vi "Boolean Counter.vi"(1 "Input Boolean":bool, 2 "Min of array which must be true":i16=5, 3 "Array Size":i32=5) -> (0 "Output Boolean":bool)   [LabVIEW 2015]
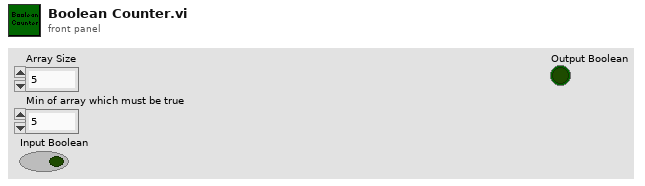
[diagram p1: front panel]
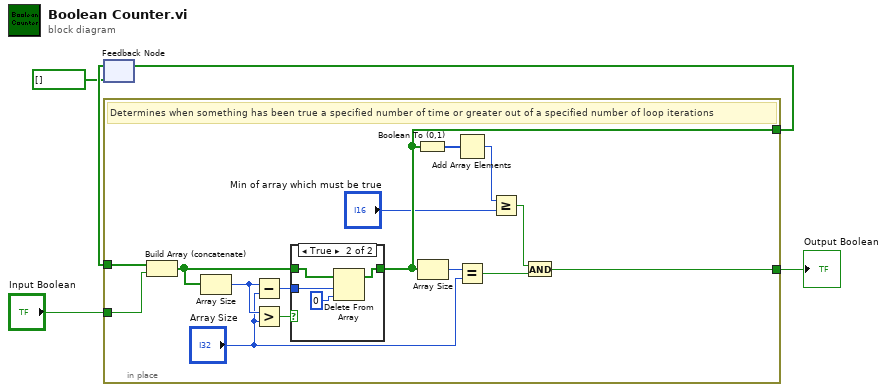
[diagram p0: block diagram]
diagram:
  n1 = feedback #1(bool[] []) -> (w4:bool[])
  n2 = in-place {
    in-place-border: w4 -> [w20]
    in-place-border: [w10] -> w5
    in-place-border: [w12] -> w1
    in-place-border: "Input Boolean" -> [w11]
    # "Determines when something has been true a specified number of time or greater out of a specified number of loop iterations"
    n3 = Build Array (concatenate)(w20, w11) -> (w19:bool[])
    n4 = Array Size(array=w19) -> (size(s)=w17:i32)
    n5 = Subtract(x=w17, y="Array Size") -> (x-y=w16:i32)
    n6 = Greater?(x=w17, y="Array Size") -> (0:w18:bool)
    n7 = case shown="True" w18 {
      tunnel: w19 -> [w21 w25]
      tunnel: [w21 w24] -> w10
      tunnel: w16 -> [_ w23]
      frame False {
      }
      frame True {
        n8 = Delete From Array(array=w25, length=w23, index=0) -> (array with subset deleted=w24:bool[])  [unwired: 1 out]
      }
    }
    n9 = Boolean To (0,1)(Boolean=w10) -> (0, 1=w9:i16[])
    n10 = Array Size(array=w10) -> (size(s)=w13:i32)
    n11 = Add Array Elements(numeric array=w9) -> (sum=w8:i16)
    n12 = Equal?(x=w13, y="Array Size") -> (x = y?=w14:bool)
    n13 = Greater Or Equal?(x=w8, y="Min of array which must be true") -> (x >= y?=w6:bool)
    n14 = And(x=w6, y=w14) -> (x .and. y?=w12:bool)
  }
  "Output Boolean" <- w1
  n15 = feedback-in #1(w5) -> ()
